vi "Get Channel Data.vi"(8 "error in":errorcluster, 9 "Count (0: Read All)":i32, 10 "index":i32, 11 "Channel in":refnum<k20>) -> (0 "error out":errorcluster, 2 "Signal":dbl[](array[numeric]), 3 "Channel out":refnum<k20>)   [LabVIEW 2017, in "Engine Simulation Toolkit System Explorer.lvlib" / "File Interface.lvlib"]
uses:
  File Interface.lvlib
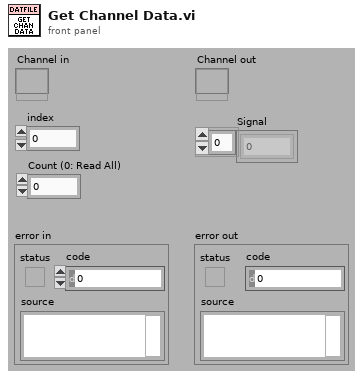
[diagram p1: front panel]
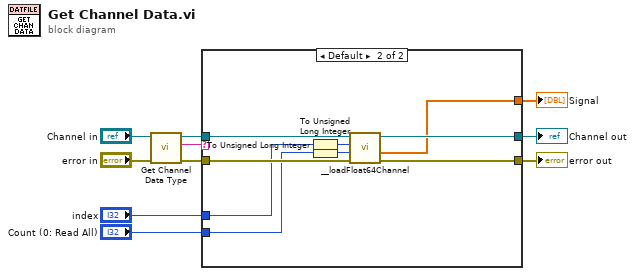
[diagram p0: block diagram]
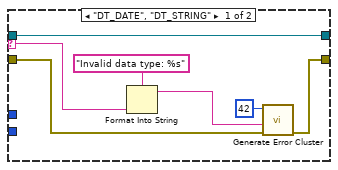
[diagram p2: hidden frame]
diagram:
  n1 = call "Get Channel Data Type.vi"("error in"="error in", "Channel in"="Channel in") -> ("error out"=w4:errorcluster, "Data Type"=w2:string, "Channel out"=w5:refnum<k20>)  [unwired: 6 in, 1 out]
  n2 = case shown="Default" w2 {
    selector: w2 -> [w14 _]
    tunnel: [w17 w20] -> w10
    tunnel: [_ w19] -> w9
    tunnel: [w12 w18] -> w8
    tunnel: w5 -> [w17 w25]
    tunnel: w4 -> [w11 w26]
    tunnel: "index" -> [_ w24]
    tunnel: "Count (0: Read All)" -> [_ w21]
    frame "DT_DATE", "DT_STRING" {
      n3 = Format Into String(format string="Invalid data type: %s", w14) -> (resulting string=w13:string)  [unwired: 2 in, 1 out]
      n4 = call "Generate Error Cluster.vi"("error in (no error)"=w11, "Additional Message"=w13, "Code"=42) -> ("error out"=w12:errorcluster)  [unwired: 8 in]
    }
    frame Default {
      n5 = To Unsigned Long Integer(number=w24) -> (unsigned 32bit integer=w23:u32)
      n6 = To Unsigned Long Integer(number=w21) -> (unsigned 32bit integer=w22:u32)
      n7 = call <vilib>:"__loadFloat64Channel.vi"("error in (no error)"=w26, "Count"=w22, "Index"=w23, "Data object in"=w25) -> ("error out"=w18:errorcluster, "Values"=w19:dbl[], "Data object out"=w20:refnum<k20>)  [unwired: 1 out]
    }
  }
  "Channel out" <- w10
  "Signal" <- w9
  "error out" <- w8
